vi "Automation_original.vi"() -> ()   [LabVIEW 2018]
uses:
  <vilib>/Utility/error.llb/DialogType.ctl
  cb6d7afe-07a1-4717-8708-8a88368bf63c.vi
panel:
  out "Min":dbl
  out "Sec":dbl
  out "H":dbl
  in  "Stop Button":bool
  out "P x Lambda Graph":cluster{dbl[], dbl[]}(graph)
  out "Corrente Atual (mA)":dbl
  out "P x I Graph":cluster{dbl[], dbl[]}(graph)
  in  "Start Button":bool
  in  "Cluster de Dados de Entrada":T1={"Corrente Inicial (mA)"=40.0, "Limite de Temperatura"=27.0, "Temperatura"=25.0, "Corrente Limite (mA)"=300, "Centralizar pico (nm)"=1550.0, "Valor de Span (nm)"=100.0, "Passo (mA)"=5.0, "Corrente Final (mA)"=110.0, "Resolucao"=enum."Normal"} {"Corrente Final (mA)" min=0.0 step=1.0; "Passo (mA)" min=1.0 step=1.0; "Valor de Span (nm)" min=0.1 max=1400.0 format="%.2f"; "Centralizar pico (nm)" format="%.2f"; "Temperatura" min=-100.0 max=199.9 step=0.1; "Limite de Temperatura" min=-100.0 max=199.9 step=0.1; "Corrente Inicial (mA)" min=0.0 step=1.0}
  out "XY Graph":T2(graph)
  in  "Pasta Destino":path=path "d:/Users/Stinky/Documents/11.04.2019/aquisicao14_HR_4mA_151_500"
  in  "GPIB Analisador de Espectros":refnum<visa-resource-name>="Advantest_Spectrometer_82357A"
  in  "GPIB Controlador Laser Diodo":refnum<visa-resource-name>="DiodeLaserController__82357A"
  in  "error in (no error)":errorcluster
  out "error out":errorcluster
  # "Tempo Gasto"
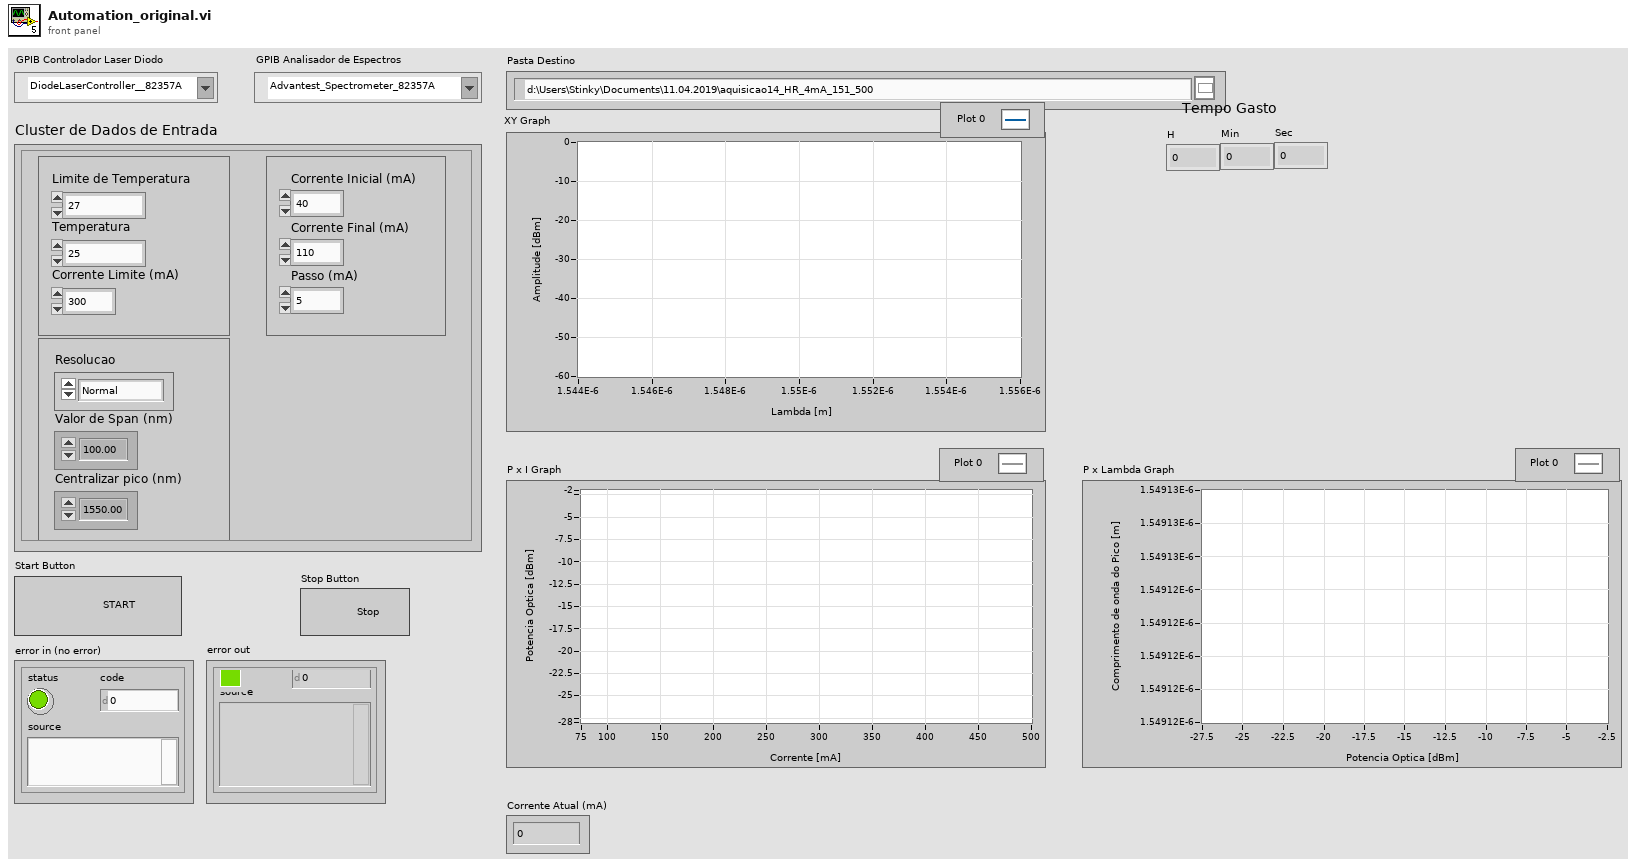
[diagram p1: front panel]
types:
  T1 = cluster{"Corrente Inicial (mA)":dbl, "Limite de Temperatura":dbl, "Temperatura":dbl, "Corrente Limite (mA)":i32, "Centralizar pico (nm)":dbl, "Valor de Span (nm)":dbl, "Passo (mA)":dbl, "Corrente Final (mA)":dbl, "Resolucao":enum16{"Normal", "High"}}
  T2 = cluster{"Wavelike Data":dbl[], "Wavelike Data":dbl[]}
  T3 = typedef "DialogType.ctl" = u16
  T4 = cluster{"Limite de Temperatura":dbl, "Temperatura":dbl, "Corrente Inicial (mA)":dbl, "Corrente Limite (mA)":i32, "Resolucao":enum16{"Normal", "High"}, "Centralizar pico (nm)":dbl, "Valor de Span (nm)":dbl}
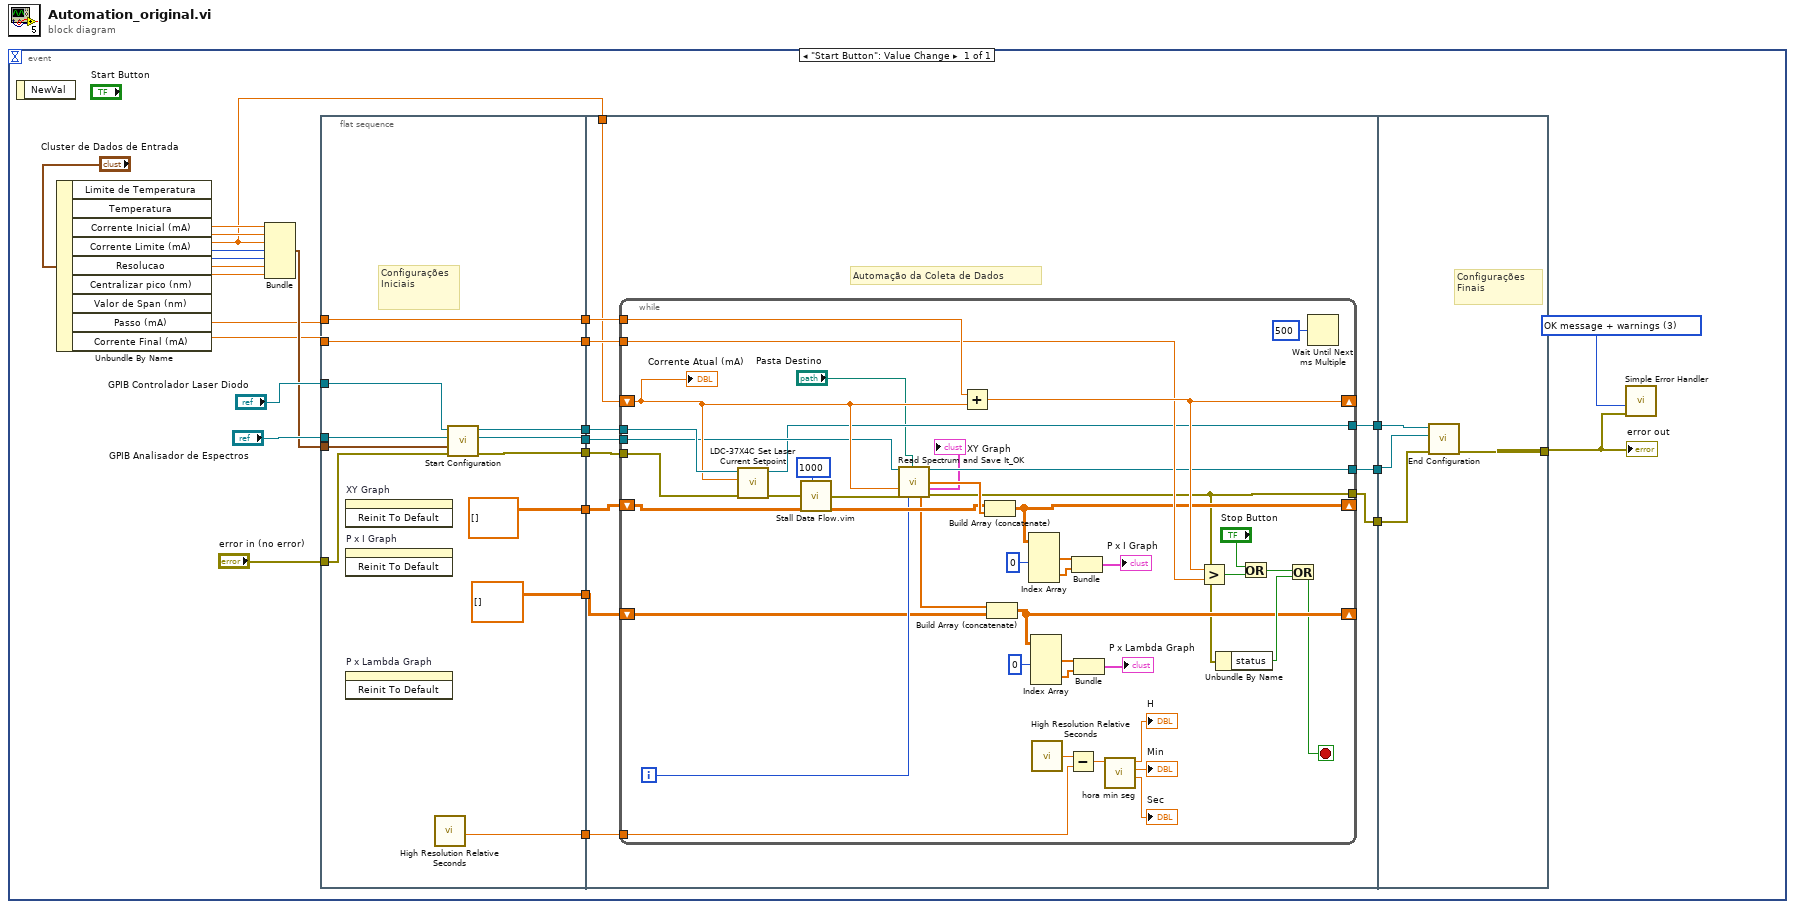
[diagram p0: block diagram]
diagram:
  n1 = event shown="[0] \"Start Button\": Value Change" {
    selector: _ -> [_]
    dyn-events: _ -> [_]
    timeout: _ -> [_]
    event "Start Button": Value Change {
      w3 = T3 3 items=["no dialog", "OK message", "continue or stop message", "OK message + warnings", "continue/stop + warnings"] ("type of dialog (OK msg:1)")
      n2 = event-data() -> ()  [unwired: 1 in, 1 out]
      n3 = Unbundle By Name("Cluster de Dados de Entrada") -> ("Limite de Temperatura"=w17:dbl, "Temperatura"=w16:dbl, "Corrente Inicial (mA)"=w8:dbl, "Corrente Limite (mA)"=w15:i32, "Resolucao"=w14:enum16{"Normal", "High"}, "Centralizar pico (nm)"=w13:dbl, "Valor de Span (nm)"=w11:dbl, "Passo (mA)"=w10:dbl, "Corrente Final (mA)"=w9:dbl)
      n4 = Bundle("Limite de Temperatura"=w17, "Temperatura"=w16, "Corrente Inicial (mA)"=w8, "Corrente Limite (mA)"=w15, "Resolucao"=w14, "Centralizar pico (nm)"=w13, "Valor de Span (nm)"=w11) -> (w12:T4)  [unwired: 1 in]
      n5 = flat-sequence {
        tunnel: "error in (no error)" -> [w30]
        tunnel: [w39] -> w27
        tunnel: [w38] -> w26
        tunnel: "GPIB Controlador Laser Diodo" -> [w37]
        tunnel: "GPIB Analisador de Espectros" -> [w36]
        tunnel: [w35] -> w25
        tunnel: [w34] -> w24
        tunnel: w10 -> [w34]
        tunnel: w9 -> [w33]
        tunnel: [w33] -> w23
        tunnel: w12 -> [w32]
        tunnel: [dbl[][] []] -> w7
        tunnel: [dbl[][] []] -> w2
        tunnel: [w28] -> w1
        tunnel: w27 -> [w51]
        tunnel: w26 -> [w50]
        tunnel: w25 -> [w49]
        tunnel: [w48] -> w22
        tunnel: w24 -> [w47]
        tunnel: w23 -> [w46]
        tunnel: w8 -> [w45]
        tunnel: w7 -> [w44]
        tunnel: [w43] -> w6
        tunnel: [w42] -> w5
        tunnel: w2 -> [w41]
        tunnel: w1 -> [w40]
        tunnel: [w97] -> w4
        tunnel: w22 -> [w96]
        tunnel: w6 -> [w95]
        tunnel: w5 -> [w94]
        frame #0 {
          # "Configurações\nIniciais"
          n6 = invoke on="XY Graph" class="XYGraph (strict)" method="Reinit To Default"() -> ()  [unwired: 3 in, 3 out]
          n7 = invoke on="P x I Graph" class="XYGraph (strict)" method="Reinit To Default"() -> ()  [unwired: 3 in, 3 out]
          n8 = invoke on="P x Lambda Graph" class="XYGraph (strict)" method="Reinit To Default"() -> ()  [unwired: 3 in, 3 out]
          n9 = call <vilib>:"High Resolution Relative Seconds.vi"() -> ("relative seconds"=w28:dbl)
          n10 = call "Start Configuration.vi"("error in (no error)"=w30, "Cluster de Dados"=w32, "GPIB Espectrometro"=w36, "GPIB Controlador Laser Diodo"=w37) -> ("error out"=w39:errorcluster, "Spectrometer out"=w35:refnum<visa-resource-name>, "Controller out"=w38:refnum<visa-resource-name>)  [unwired: 5 in]
        }
        frame #1 {
          # "Automação da Coleta de Dados"
          n11 = while {
            shift-right: [w87] -> _
            shift-left: w45 -> [w88]
            tunnel: w51 -> [w80]
            tunnel: w50 -> [w93]
            tunnel: w49 -> [w86]
            tunnel: [w83] -> w48
            tunnel: w47 -> [w85]
            tunnel: w46 -> [w84]
            shift-right: [w77] -> _
            shift-left: w44 -> [w78]
            tunnel: [w62] -> w43
            tunnel: [w71] -> w42
            shift-right: [w63] -> _
            shift-left: w41 -> [w64]
            tunnel: w40 -> [w57]
            i -> [w72]
            stop <- w59 stop-if-true
            n12 = call "LDC-37X4C Set Laser Current Setpoint.vi"("error in (no error)"=w80, "Current"=w88, "VISA resource name"=w93) -> ("error out"=w91:errorcluster, "VISA resource name out"=w83:refnum<visa-resource-name>)  [unwired: 7 in]
            n13 = call "Stall Data Flow.vim"("value in"=w91, "milliseconds to wait"=u32 1000) -> ("value out"=w89:errorcluster)  [unwired: 1 out]
            n14 = call "Read Spectrum and Save It_OK.vi"("VISA Session"=w86, "Pasta Destino DESTA aquisicao"="Pasta Destino", "Corrente Atual (mA)"=w88, "Error In"=w89, "Iteracao"=w72) -> ("Copy VISA Session"=w71:refnum<visa-resource-name>, "PxI"=w79:dbl[], "XY Graph"=→"XY Graph":T2, "PxLambda"=w65:dbl[], "Error Out"=w62:errorcluster)  [unwired: 4 in, 2 out]
            n15 = Add(x=w85, y=w88) -> (x+y=w87:dbl)
            n16 = Build Array (concatenate)(w78, w79) -> (w77:dbl[][])
            n17 = Build Array (concatenate)(w65, w64) -> (w63:dbl[][])
            n18 = Index Array(array=w77, index (col) #1=0 ("disabled index (col)")) -> (element #1=w75:dbl[], element #2=w74:dbl[])  [unwired: 3 in]
            n19 = Index Array(array=w63, index (col) #1=0 ("disabled index (col)")) -> (element #1=w68:dbl[], element #2=w67:dbl[])  [unwired: 3 in]
            n20 = call <vilib>:"High Resolution Relative Seconds.vi"() -> ("relative seconds"=w58:dbl)
            n21 = Subtract(x=w58, y=w57) -> (x-y=w56:dbl)
            n22 = Bundle(w75, w74) -> (→"P x I Graph":cluster{dbl[], dbl[]})  [unwired: 1 in]
            n23 = Bundle(w68, w67) -> (→"P x Lambda Graph":cluster{dbl[], dbl[]})  [unwired: 1 in]
            n24 = call "hora min seg.vi"("Total time in seconds"=w56) -> ("Sec"=→"Sec":dbl, "Min"=→"Min":dbl, "H"=→"H":dbl)  [unwired: 8 in]
            n25 = Greater?(x=w87, y=w84) -> (0:w90:bool)
            n26 = Unbundle By Name(w62) -> ("status"=w81:bool)
            n27 = Or(x="Stop Button", y=w90) -> (x .or. y?=w82:bool)
            n28 = Or(x=w82, y=w81) -> (x .or. y?=w59:bool)
            n29 = Wait Until Next ms Multiple(millisecond multiple=u32 500) -> ()  [unwired: 1 out]
            "Corrente Atual (mA)" <- w88
          }
        }
        frame #2 {
          # "Configurações\nFinais"
          n30 = call "End Configuration.vi"("error in (no error)"=w95, "GPIB Espectrometro"=w94, "GPIB Controlador Laser Diodo"=w96) -> ("error out"=w97:errorcluster)  [unwired: 8 in]
        }
      }
      n31 = call <vilib>:"Simple Error Handler.vi"("type of dialog (OK msg:1)"=w3, "error in (no error)"=w4) -> ()  [unwired: 3 in, 5 out]
      "error out" <- w4
    }
  }
